vi "Clear Multiple listbox.vi"(8 "error in (no error)":errorcluster, 11 "Listbox Reference In":refnum<vi>) -> (0 "error out":errorcluster, 3 "Listbox Reference Out":refnum<vi>)   [LabVIEW 2024]
doc: "Clears the content in the multiple listbox."
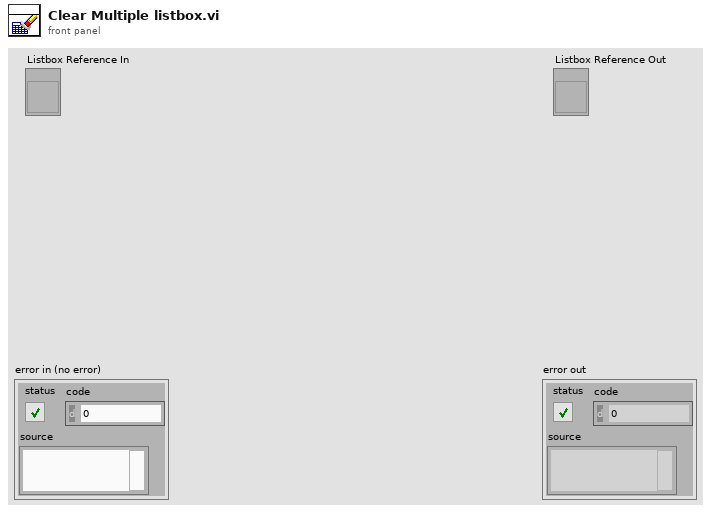
[diagram p1: front panel]
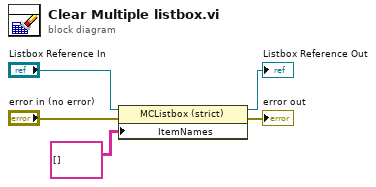
[diagram p0: block diagram]
diagram:
  n1 = property class="MCListbox (strict)"(reference="Listbox Reference In", error in="error in (no error)", "ItemNames"=string[][] [] ("Item Names")) -> (reference out=→"Listbox Reference Out":refnum<vi>, error out=→"error out":errorcluster)
